vi "Configure LIST Status.vi"(8 "error in (no error)":errorcluster, 9 "Status (T: Enable)":bool=TRUE, 10 "Sweep Point":i32=1 min=1 max=10 step=1, 11 "VISA resource name":refnum<visa-resource-name>) -> (0 "error out":errorcluster, 3 "VISA resource name out":refnum<visa-resource-name>)   [LabVIEW 2014, in "LCR Meter.lvlib"]
doc: "Turns on/off the specified sweep point."
uses:
  <instrlib>/LCR Meter/Examples/LCR Meter Acquire Single_1 Folder/LCR Meter.lvlib
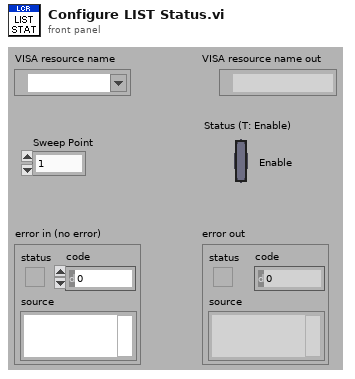
[diagram p1: front panel]
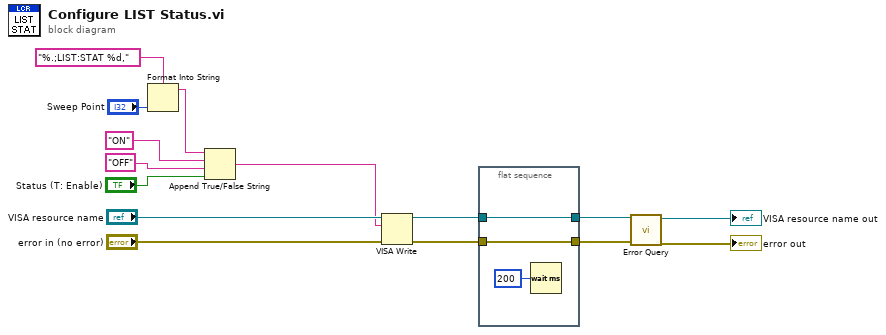
[diagram p0: block diagram]
diagram:
  n1 = Format Into String(format string="%.;LIST:STAT %d,", "Sweep Point") -> (resulting string=w2:string)  [unwired: 2 in, 1 out]
  n2 = Append True/False String(1:"Status (T: Enable)", 2:"OFF" ("false string"), 3:"ON" ("true string"), 4:w2) -> (0:w1:string)
  n3 = VISA Write(VISA resource name="VISA resource name", write buffer=w1, error in (no error)="error in (no error)") -> (VISA resource name out=w11:refnum<visa-resource-name>, error out=w9:errorcluster)  [unwired: 1 out]
  n4 = flat-sequence {
    tunnel: w11 -> [w18]
    tunnel: [w18] -> w10
    tunnel: w9 -> [w17]
    tunnel: [w17] -> w8
    frame #0 {
      n5 = Wait (ms)(milliseconds to wait=u32 200) -> ()  [unwired: 1 out]
    }
  }
  n6 = call <instrlib>:"Error Query.vi"("error in (no error)"=w8, "VISA resource name"=w10) -> ("error out"=→"error out":errorcluster, "VISA resource name out"=→"VISA resource name out":refnum<visa-resource-name>)  [unwired: 6 in, 2 out]
